vi "Alm.vi"(8 "error in (no error)":errorcluster caption="错误输入（无错误）", 11 "AllControls Out":T1) -> ()   [LabVIEW 2017]
uses:
  Ctrls/AllControls.ctl
  ComVIS/_OpenG/comparison/comparison.llb/1D Boolean Array Changed__ogtk.vi
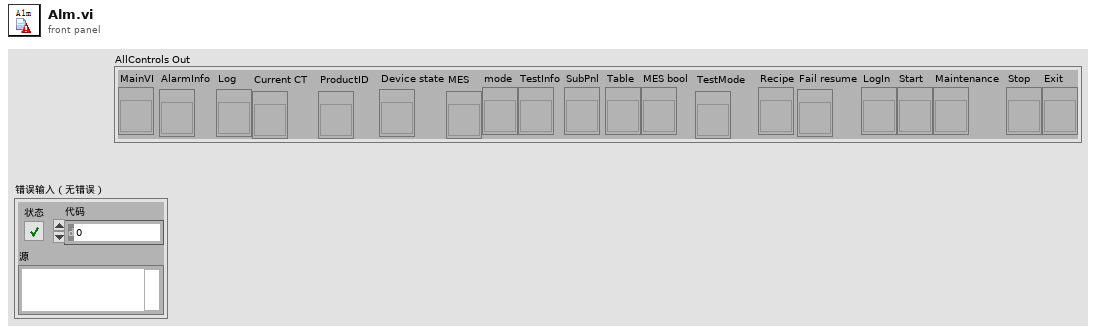
[diagram p1: front panel]
types:
  T1 = typedef "AllControls.ctl" = cluster{"MainVI":refnum<vi>, "AlarmInfo":refnum<vi>, "Log":refnum<vi>, "Current CT":refnum<vi>, "ProductID":refnum<vi>, "Device state":refnum<vi>, "MES":refnum<vi>, "mode":refnum<vi>, "TestInfo":refnum<vi>, "SubPnl":refnum<vi>, "Table":refnum<vi>, "MES bool":refnum<vi>, "TestMode":refnum<vi>, "Recipe":refnum<vi>, "Fail resume":refnum<vi>, "LogIn":refnum<vi>, "Start":refnum<vi>, "Maintenance":refnum<vi>, "Stop":refnum<vi>, "Exit":refnum<vi>}
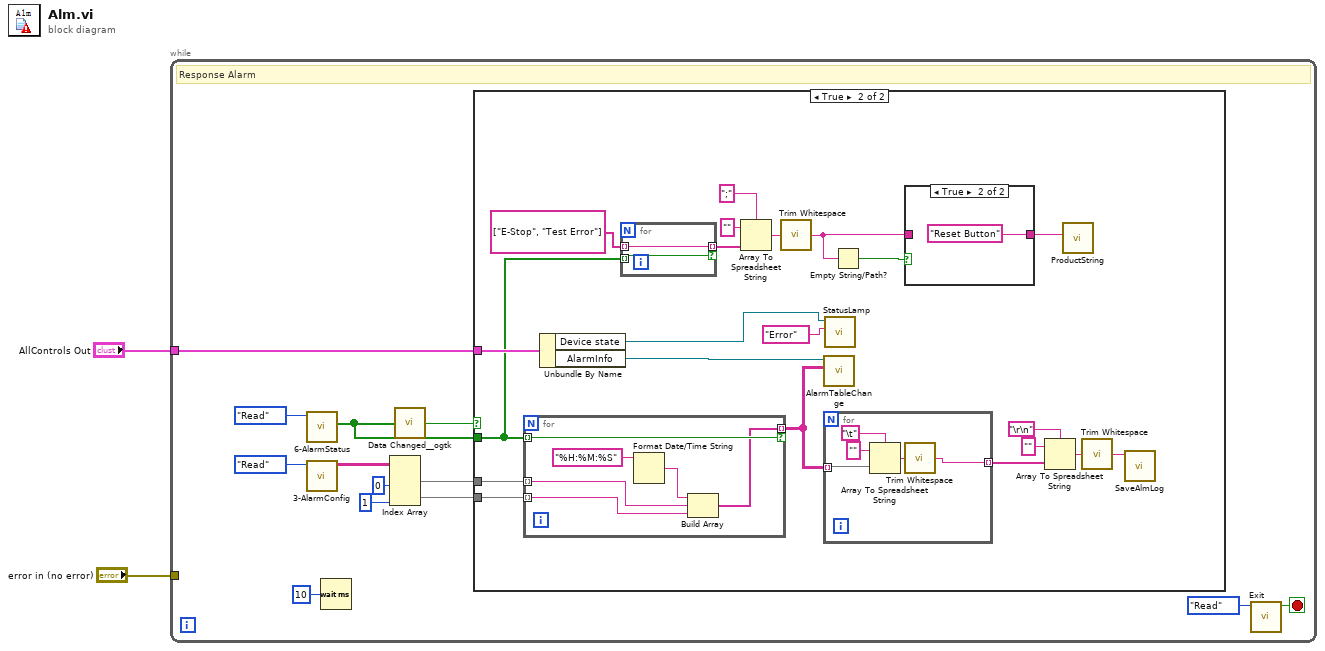
[diagram p0: block diagram]
diagram:
  n1 = while {
    tunnel: "AllControls Out" -> [w12]
    tunnel: "error in (no error)" -> [_]
    stop <- w15 stop-if-true
    # "Response Alarm"
    n2 = call "6-AlarmStatus.vi"("Step"=enum16{"Initial", "Write", "Read"}."Read") -> ("AlarmValue Out"=w4:bool[])  [unwired: 9 in, 1 out]
    n3 = call "3-AlarmConfig.vi"("Step"=enum16{"Initial", "Write", "Read"}."Read") -> ("AlarmConfig Out"=w9:string[][])  [unwired: 9 in, 1 out]
    n4 = Wait (ms)(milliseconds to wait=u32 10 ("等待时间（毫秒）")) -> ()  [unwired: 1 out]
    n5 = Index Array(array=w9, index (col) #1=0 ("禁用的索引 (列)"), index (col) #2=1 ("索引 (列)")) -> (element #1=w6:string[], element #2=w5:string[])  [unwired: 2 in]
    n6 = call-poly "Data Changed__ogtk.vi"("1D Boolean Array"=w4) -> ("Changed"=w3:bool)
    n7 = case shown="True" w3 {
      tunnel: w6 -> [_ w36]
      tunnel: w5 -> [_ w35]
      tunnel: w4 -> [_ w24]
      tunnel: w12 -> [_ w34]
      frame False {
      }
      frame True {
        n8 = for {
          tunnel: w36 -> [w49] mode=indexing
          tunnel: w35 -> [w48] mode=indexing
          tunnel: w24 -> [w47] mode=indexing
          tunnel: [w46] -> w28 mode=indexing if=w47
          n9 = Format Date/Time String(time format string (%c)="%H:%M:%S" ("时间格式字符串(%c)")) -> (date/time string=w50:string)  [unwired: 2 in]
          n10 = Build Array(w50, w49, w48) -> (w46:string[])
        }
        n11 = Unbundle By Name(w34) -> ("Device state"=w25:refnum<vi>, "AlarmInfo"=w29:refnum<vi>)
        n12 = for {
          tunnel: w24 -> [w39] mode=indexing
          tunnel: [w40] -> w22 mode=indexing if=w39
          tunnel: string[] ["E-Stop", "Test Error"] -> [w40] mode=indexing
        }
        n13 = Array To Spreadsheet String(delimiter (Tab)=";", array=w22, 3:"" ("format string")) -> (spreadsheet string=w19:string)
        n14 = call <vilib>:"Trim Whitespace.vi"("string"=w19) -> ("trimmed string"=w18:string)  [unwired: 1 in]
        n15 = call "AlarmTableChange.vi"("AlarmData"=w28, "AlarmInfo"=w29) -> ()  [unwired: 9 in, 1 out]
        n16 = for {
          tunnel: w28 -> [w45] mode=indexing
          tunnel: [w41] -> w31 mode=indexing
          n17 = Array To Spreadsheet String(delimiter (Tab)="\t", array=w45, 3:"" ("format string")) -> (spreadsheet string=w42:string)
          n18 = call <vilib>:"Trim Whitespace.vi"("string"=w42) -> ("trimmed string"=w41:string)  [unwired: 1 in]
        }
        n19 = call "StatusLamp.vi"("State"="Error", "Boolean输入"=w25) -> ()  [unwired: 9 in, 1 out]
        n20 = Empty String/Path?(string/path=w18) -> (empty?=w17:bool)
        n21 = case shown="True" w17 {
          tunnel: w18 -> [w37 _]
          tunnel: [w37 "Reset Button" ("值")] -> w16
          frame False {
          }
          frame True {
          }
        }
        n22 = Array To Spreadsheet String(delimiter (Tab)="\r\n", array=w31, 3:"" ("format string")) -> (spreadsheet string=w30:string)
        n23 = call "ProductString.vi"("String"=w16) -> ()  [unwired: 10 in, 1 out]
        n24 = call <vilib>:"Trim Whitespace.vi"("string"=w30) -> ("trimmed string"=w27:string)  [unwired: 1 in]
        n25 = call "SaveAlmLog.vi"("AlmLog"=w27) -> ()  [unwired: 10 in, 1 out]
      }
    }
    n26 = call "Exit.vi"("Step"=enum16{"Initial", "Write", "Read"}."Read" ("step")) -> ("Exit Out"=w15:bool)  [unwired: 9 in, 1 out]
  }
